vi "array - rotate - col.vi"(4 "rotate column":i32, 11 "input matrix":T1) -> (3 "output matrix":T1)   [LabVIEW 2021]
uses:
  <vilib>/Analysis/Matrix/Datatypes/ComplexMatrix.ctl
  <vilib>/Analysis/Matrix/NI_Matrix.lvlib
panel:
  out "x-y*floor(x/y)":i32
  in  "dim":i32
  in  "rotate row":i32
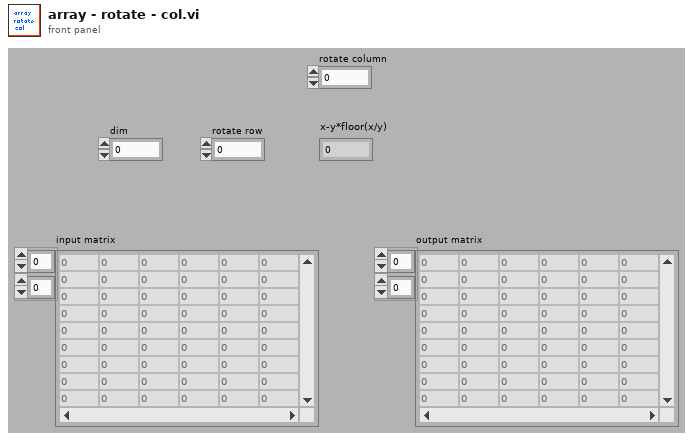
[diagram p1: front panel]
types:
  T1 = typedef "NI_Matrix.lvlib/ComplexMatrix.ctl" = cdb[][]
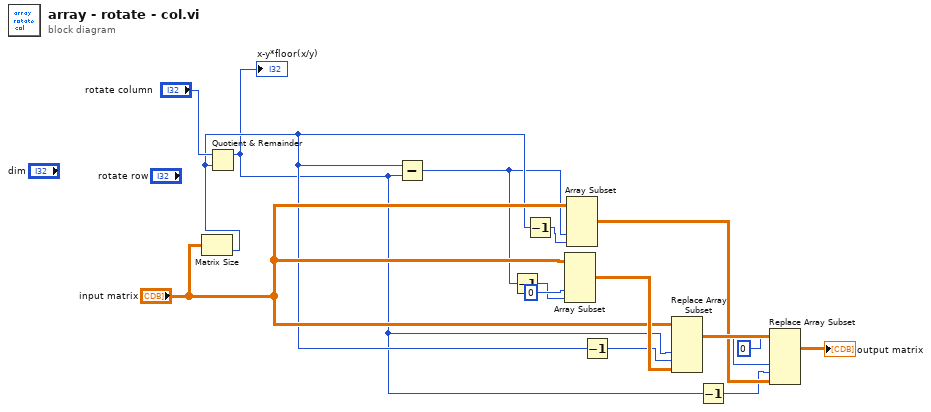
[diagram p0: block diagram]
diagram:
  n1 = Matrix Size(0:"input matrix") -> (2:w9:i32)  [unwired: 1 out]
  n2 = Quotient & Remainder(x="rotate column", y=w9) -> (x-y*floor(x/y)=w4:i32)  [unwired: 1 out]
  "x-y*floor(x/y)" <- w4
  n3 = Subtract(x=w9, y=w4) -> (x-y=w8:i32)
  n4 = Decrement(x=w8) -> (x-1=w5:i32)
  n5 = Decrement(x=w9) -> (x-1=w7:i32)
  n6 = Array Subset(array="input matrix", index (col)=0 ("row 1"), length (col)=w5) -> (w15:T1)  [unwired: 2 in]
  n7 = Array Subset(array="input matrix", index (col)=w8, length (col)=w7) -> (w12:T1)  [unwired: 2 in]
  n8 = Decrement(x=w9) -> (x-1=w3:i32)
  n9 = Replace Array Subset(array="input matrix", new element=w15, index (dim 2)=w4, index (dim 3)=w3) -> (w14:T1)  [unwired: 2 in]
  n10 = Decrement(x=w4) -> (x-1=w1:i32)
  n11 = Replace Array Subset(array=w14, new element=w12, index (dim 2)=0 ("row 1"), index (dim 3)=w1) -> (→"output matrix":T1)  [unwired: 2 in]
